vi "Pickering 40-295 System Explorer.vi"(8 "error in (no error)":errorcluster, 11 "Node Ptr":T1 format="%.0x") -> (0 "error out":errorcluster)   [LabVIEW 2014, in "Pickering 40-295.lvlib"]
uses:
  Pickering 40-295.lvlib
  <vilib>/NI Veristand/Custom Device API/Custom Device Item Ref.ctl
  <vilib>/NI Veristand/Custom Device API/Get Item Property (String).vi
  <vilib>/NI Veristand/Custom Device API/Set Item Property (String).vi
  <vilib>/NI Veristand/Custom Device API/Custom Device API.lvlib
panel:
  in  "Header 2":cluster{"Section Name":string}={"Section Name"="Pickering 40-295 Hardware Settings"}
  in  "Board Resource Name":string
  in  "Header":cluster{"Section Name":string}={"Section Name"="Pickering 40-295 Device Settings"}
  in  "Description":string
  in  "Name":string
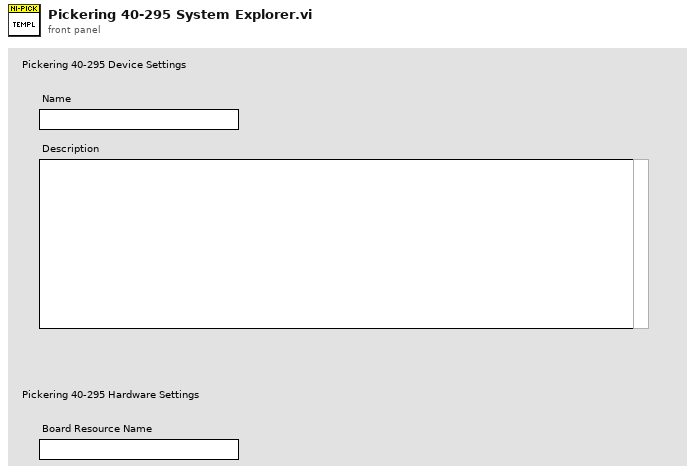
[diagram p1: front panel]
types:
  T1 = typedef "Custom Device API.lvlib/Custom Device Item Ref.ctl" = u64
  T2 = typedef "Custom Device API.lvlib/Custom Device Item Info.ctl" = cluster{"Name":string, "Is Channel":bool, "GUID":string, "Is Waveform":bool}
  T3 = typedef "Custom Device API.lvlib/Custom Device Commands.ctl" = enum16{"Default", "Item renamed", "Shutdown", "Dynamic button pressed"}
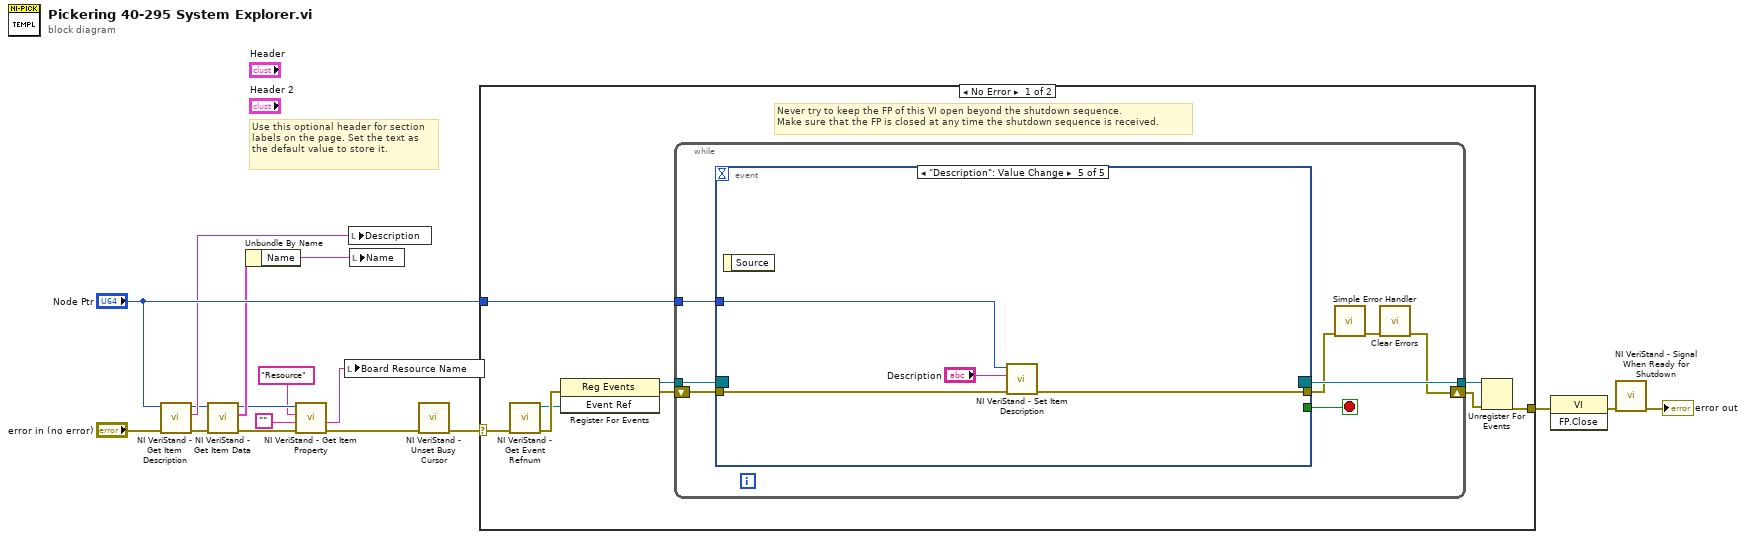
[diagram p0: block diagram]
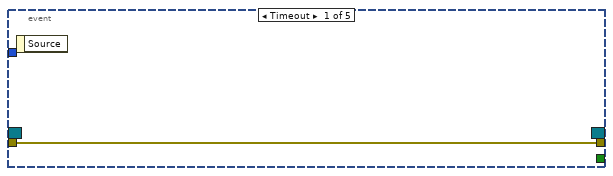
[diagram p2: hidden frame]
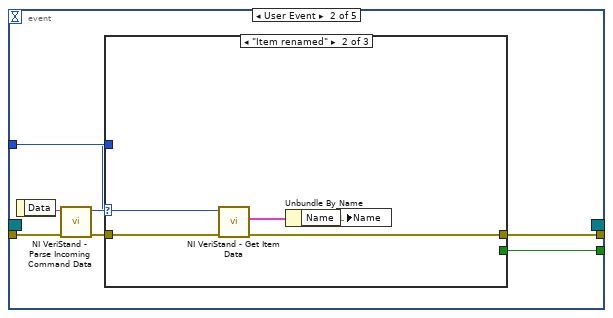
[diagram p3: hidden frame]
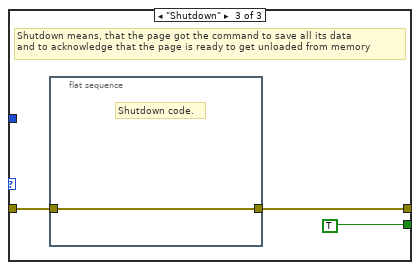
[diagram p5: hidden frame]
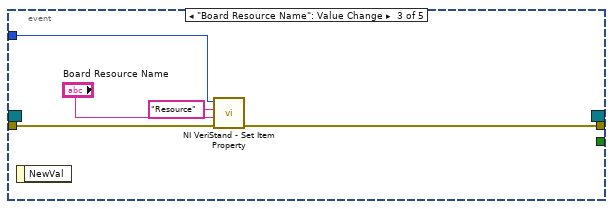
[diagram p6: hidden frame]
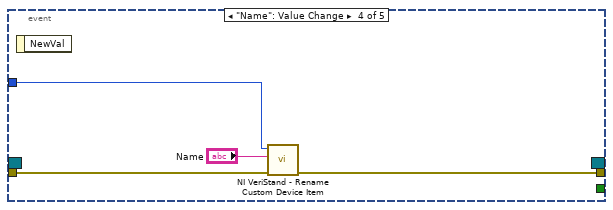
[diagram p7: hidden frame]
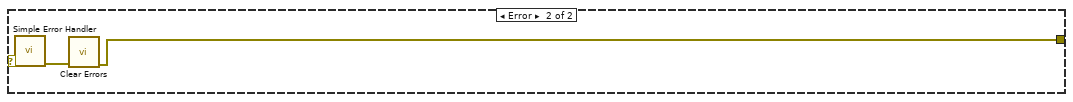
[diagram p8: hidden frame]
diagram:
  # "Use this optional header for section labels on the page. Set the text as the default value to store it."
  n1 = call <vilib>:"NI VeriStand - Get Item Description.vi"("error in (no error)"="error in (no error)", "Item Ref in"="Node Ptr") -> ("error out"=w10:errorcluster, "Description"=w11:string, "Item Ref out"=w9:T1)  [unwired: 7 out]
  n2 = call <vilib>:"NI VeriStand - Get Item Data.vi"("error in (no error)"=w10, "Item Ref in"=w9) -> ("error out"=w6:errorcluster, "Item Info"=w8:T2, "Item Ref out"=w4:T1)  [unwired: 7 out]
  n3 = Unbundle By Name(w8) -> ("Name"=w7:string)
  n4 = call-poly <vilib>:"NI VeriStand - Get Item Property.vi"("error in (no error)"=w6, "Default Value"="", "Property Name"="Resource", "Item Ref in"=w4) -> ("error out"=w5:errorcluster, "Value"=w1:string)  [unwired: 6 out]
  n5 = local write "Board Resource Name"(w1) -> ()
  n6 = local write "Description"(w11) -> ()
  n7 = local write "Name"(w7) -> ()
  n8 = call <vilib>:"NI VeriStand - Unset Busy Cursor.vi"("error in (no error)"=w5) -> ("error out"=w13:errorcluster)  [unwired: 10 out]
  n9 = case shown="No Error" w13 {
    selector: w13 -> [w18 w68]
    tunnel: [w23 w66] -> w17
    tunnel: "Node Ptr" -> [w19 _]
    frame No Error {
      # "Never try to keep the FP of this VI open beyond the shutdown sequence.\nMake sure that the FP is closed at any time the shutdown sequence is received."
      n10 = call <vilib>:"NI VeriStand - Get Event Refnum.vi"("error in (no error)"=w18) -> ("error out"=w26:errorcluster, "Event Ref"=w22:refnum<user-event>)  [unwired: 9 out]
      n11 = register-events(error in=w26, w22) -> (reference out=w20:refnum<event-registration>, error out=w21:errorcluster)  [unwired: 1 in]
      n12 = while {
        tunnel: [w34] -> w25
        tunnel: w20 -> [w32]
        tunnel: w19 -> [w30]
        shift-right: [w27] -> w24
        shift-left: w21 -> [w33]
        stop <- w31 stop-if-true
        n13 = event shown="[4] \"Description\": Value Change" {
          selector: w32 -> [_ _ _ _ _]
          dyn-events: [_ _ _ _ _] -> w34
          timeout: _ -> [_ _ _ _ _]
          tunnel: w33 -> [w35 w42 w57 w61 w64]
          tunnel: [_ w38 _ _ _] -> w31
          tunnel: [w35 w37 w53 w60 w63] -> w29
          tunnel: w30 -> [_ w36 w55 w59 w65]
          event Timeout {
            n14 = event-data() -> ()  [unwired: 2 out]
          }
          event User Event {
            n15 = event-data() -> ("Data"=w41:string)  [unwired: 1 out]
            n16 = call <vilib>:"NI VeriStand - Parse Incoming Command Data.vi"("error in (no error)"=w42, "Incoming data"=w41) -> ("error out"=w40:errorcluster, "Action"=w39:T3)  [unwired: 8 out]
            n17 = case shown="\"Item renamed\"" w39 {
              tunnel: w40 -> [w43 w48 w50]
              tunnel: [_ _ TRUE] -> w38
              tunnel: [w43 w45 w49] -> w37
              tunnel: w36 -> [_ w47 _]
              frame "Default", Default {
              }
              frame "Item renamed" {
                n18 = call <vilib>:"NI VeriStand - Get Item Data.vi"("error in (no error)"=w48, "Item Ref in"=w47) -> ("error out"=w45:errorcluster, "Item Info"=w46:T2)  [unwired: 8 out]
                n19 = Unbundle By Name(w46) -> ("Name"=w44:string)
                n20 = local write "Name"(w44) -> ()
              }
              frame "Shutdown" {
                # "Shutdown means, that the page got the command to save all its data\nand to acknowledge that the page is ready to get unloaded from memory"
                n21 = flat-sequence {
                  tunnel: w50 -> [w52]
                  tunnel: [w52] -> w49
                  frame #0 {
                    # "Shutdown code."
                  }
                }
              }
            }
          }
          event "Board Resource Name": Value Change {
            n22 = event-data() -> ()  [unwired: 2 out]
            n23 = call-poly <vilib>:"NI VeriStand - Set Item Property.vi"("error in (no error)"=w57, "Value"="Board Resource Name", "Property Name"="Resource", "Item Ref in"=w55) -> ("error out"=w53:errorcluster)  [unwired: 7 out]
          }
          event "Name": Value Change {
            n24 = event-data() -> ()  [unwired: 2 out]
            n25 = call <vilib>:"NI VeriStand - Rename Custom Device Item.vi"("error in (no error)"=w61, "New Name"="Name", "Item Ref in"=w59) -> ("error out"=w60:errorcluster)  [unwired: 1 in, 7 out]
          }
          event "Description": Value Change {
            n26 = event-data() -> ()  [unwired: 2 out]
            n27 = call <vilib>:"NI VeriStand - Set Item Description.vi"("error in (no error)"=w64, "Description"="Description", "Item Ref in"=w65) -> ("error out"=w63:errorcluster)  [unwired: 8 out]
          }
        }
        n28 = call <vilib>:"Simple Error Handler.vi"("error in (no error)"=w29) -> ("error out"=w28:errorcluster)  [unwired: 1 in, 7 out]
        n29 = call <vilib>:"Clear Errors.vi"("error in (no error)"=w28) -> ("error out"=w27:errorcluster)  [unwired: 1 in, 5 out]
      }
      n30 = Unregister For Events(event registration refnum=w25, error in=w24) -> (error out=w23:errorcluster)
    }
    frame Error {
      n31 = call <vilib>:"Simple Error Handler.vi"("error in (no error)"=w68) -> ("error out"=w67:errorcluster)  [unwired: 1 in, 7 out]
      n32 = call <vilib>:"Clear Errors.vi"("error in (no error)"=w67) -> ("error out"=w66:errorcluster)  [unwired: 1 in, 5 out]
    }
  }
  n33 = invoke class="VI" method="FP.Close"(error in=w17) -> (error out=w16:errorcluster)  [unwired: 2 in, 2 out]
  n34 = call <vilib>:"NI VeriStand - Signal When Ready for Shutdown.vi"("error in (no error)"=w16) -> ("error out"=→"error out":errorcluster)  [unwired: 10 out]
